vi "State_Machine.vi"(8 "error in (no error)":errorcluster caption="entrée d'erreur (pas d'erreur)", 11 "Get_Voltage en entrée":refnum<class "Nodon_Generate_SN.lvclass">) -> (0 "error out":errorcluster caption="sortie d'erreur", 2 "Json_String":string, 3 "Get_Voltage en sortie":refnum<class "Nodon_Generate_SN.lvclass">)   [LabVIEW 2020, in "Library Test.lvlib" / "Nodon_Generate_SN.lvclass"]
uses:
  Nodon_Generate_SN.lvclass
  E:/Dev/SVN TB45/TB45/Class/Test/Test (Default)/Test (Default).lvclass
  Database/Database Altyor/Database Altyor.lvclass
  E:/Dev/SVN TB45/TB45/Class/Database/Database drivers/Database Drivers.lvclass
  JSON API/JSON Value/Set from JSON string.vi
  Instrument/Instrument (Default)/Class Instrument (Default).lvclass
  JSON API/JSON Value/JSON Value.lvclass
  Nodon_Generate_SN.lvclass/Nodon_Generate_SN.ctl
  JSON API/Variant JSON/Variant JSON.lvlib
  JSON API/Get Polymorphic/JSON GetSet.lvlib
  Commun VI/Library Commun.lvlib
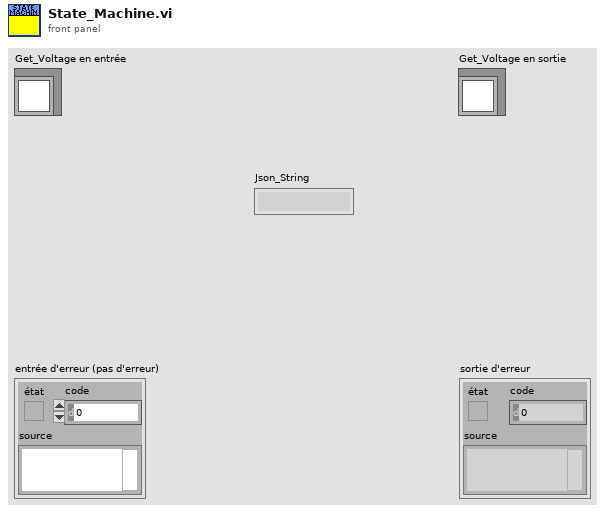
[diagram p1: front panel]
types:
  T1 = cluster{"Connection Name ODBC":string, "DatabaseName":string, "Condition":string, "Type Data ":enum16{"Data Product", "Data Test"}, "Database Altyor":refnum<class "Database Altyor.lvclass">}
  T2 = cluster{"idTest":u32, "CreationDate":string, "EndOfProduction":string, "OrderNumber":string, "Batch":string, "ProductName":string, "PartNumber":string, "SerialNumber":string, "Operator":string, "Result":string, "AdditionalInformation":string}[]
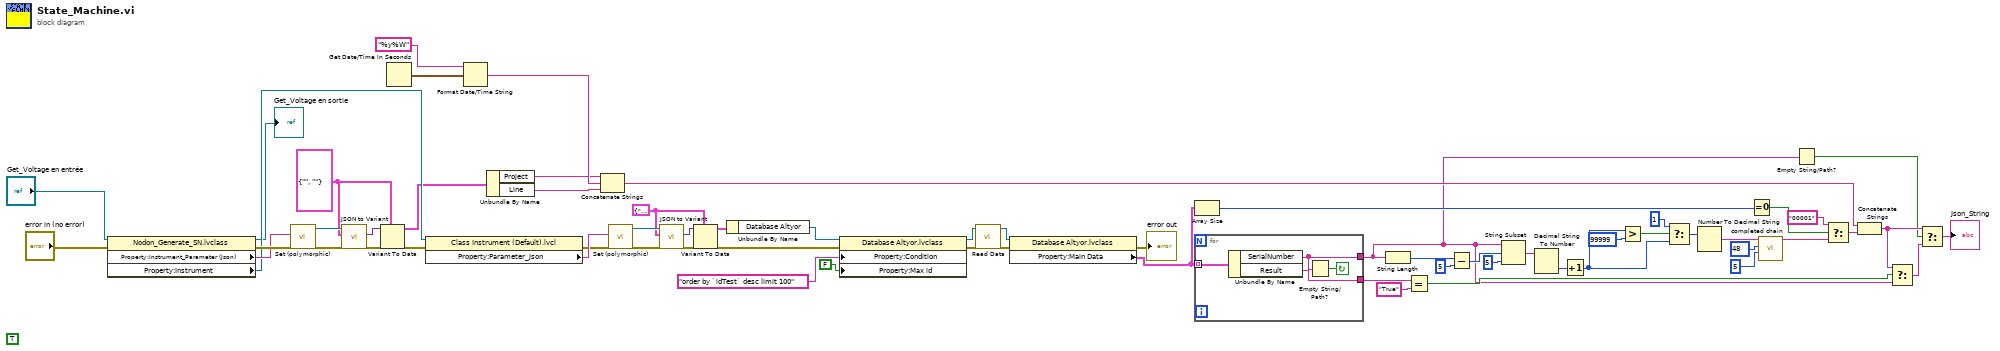
[diagram p0: block diagram]
diagram:
  (unwired) TRUE ("Max id")
  w48 = cluster{"Project":string, "Line":string} {"Project"="", "Line"=""}
  w60 = T1 {"Connection Name ODBC"="", "DatabaseName"="", "Condition"="", "Type Data "=enum."Data Product", "Database Altyor"=refnum} ("Parameter")
  n1 = property class="Nodon_Generate_SN.lvclass"(reference="Get_Voltage en entrée", error in="error in (no error)") -> (reference out=→"Get_Voltage en sortie":refnum<class "Nodon_Generate_SN.lvclass">, error out=w52:errorcluster, "Property:Instrument_Parameter (Json)"=w51:string, "Property:Instrument"=w47:refnum<class "Class Instrument (Default).lvclass">)
  n2 = call-poly "Set (polymorphic).vi"("error in (no error)"=w52, "JSON stream"=w51) -> ("error out"=w54:errorcluster, "JSON Value out"=w56:refnum<class "JSON Value.lvclass">)  [unwired: 7 in, 1 out]
  n3 = call "JSON to Variant.vi"("error in (no error)"=w54, "Variant (Data Type)"=w48, "JSON Value"=w56) -> ("error out"=w55:errorcluster, "Variant out"=w53:variant)  [unwired: 7 in]
  n4 = Variant To Data(error in=w55, type=w48, Variant=w53) -> (data=w42:cluster{"Project":string, "Line":string}, error out=w46:errorcluster)
  n5 = Get Date/Time In Seconds() -> (seconds since 1Jan1904=w45:timestamp)
  n6 = property class="Class Instrument (Default).lvcl"(reference=w47, error in=w46) -> (error out=w58:errorcluster, "Property:Parameter_Json"=w59:string)  [unwired: 1 out]
  n7 = Format Date/Time String(time format string (%c)="%y%W" ("chaîne de format de l'heure (%c)"), seconds (now)=w45) -> (date/time string=w43:string)  [unwired: 1 in]
  n8 = Unbundle By Name(w42) -> ("Project"=w41:string, "Line"=w40:string)
  n9 = Concatenate Strings(w41, w43, w40) -> (w18:string)
  n10 = call-poly "Set (polymorphic).vi"("error in (no error)"=w58, "JSON stream"=w59) -> ("error out"=w62:errorcluster, "JSON Value out"=w64:refnum<class "JSON Value.lvclass">)  [unwired: 7 in, 1 out]
  n11 = call "JSON to Variant.vi"("error in (no error)"=w62, "Variant (Data Type)"=w60, "JSON Value"=w64) -> ("error out"=w63:errorcluster, "Variant out"=w61:variant)  [unwired: 7 in]
  n12 = Variant To Data(error in=w63, type=w60, Variant=w61) -> (data=w57:T1, error out=w12:errorcluster)
  n13 = Unbundle By Name(w57) -> ("Database Altyor"=w11:refnum<class "Database Altyor.lvclass">)
  n14 = property class="Database Altyor.lvclass"(reference=w11, error in=w12, "Property:Condition"="order by `idTest` desc limit 100" ("chaîne"), "Property:Max id"=FALSE ("Max id")) -> (reference out=w23:refnum<class "Database Altyor.lvclass">, error out=w22:errorcluster)
  n15 = call-dynamic "Read Data.vi"("error in (no error)"=w22, "Database Altyor en entrée"=w23) -> ("error out"=w20:errorcluster, "Database Altyor en sortie"=w21:refnum<class "Database Altyor.lvclass">)  [unwired: 8 in]
  n16 = property class="Database Altyor.lvclass"(reference=w21, error in=w20) -> (error out=→"error out":errorcluster, "Property:Main Data"=w10:T2)  [unwired: 1 out]
  n17 = Array Size(array=w10) -> (size(s)=w9:i32)
  n18 = for {
    tunnel: w10 -> [w68] mode=indexing
    tunnel: [w67] -> w8
    tunnel: [w66] -> w2
    stop <- w65 continue-if-true
    n19 = Unbundle By Name(w68) -> ("SerialNumber"=w66:string, "Result"=w67:string)
    n20 = Empty String/Path?(string/path=w66) -> (empty?=w65:bool)
  }
  n21 = String Length(string=w2) -> (length=w38:i32)
  n22 = Equal?(x=w8, y="True") -> (x = y?=w15:bool)
  n23 = Subtract(x=w38, y=5 ("x")) -> (x-y=w37:i32)
  n24 = String Subset(string=w2, offset (0)=w37, length (rest)=5 ("longueur (reste)")) -> (substring=w31:string)
  n25 = Decimal String To Number(string=w31) -> (number=w30:i32)  [unwired: 2 in, 1 out]
  n26 = Increment(x=w30) -> (x+1=w26:i32)
  n27 = Greater?(x=w26, y=99999) -> (0:w28:bool)
  n28 = Select(t=1 ("y"), s=w28, f=w26) -> (s? t:f=w25:i32)
  n29 = Number To Decimal String(number=w25) -> (decimal integer string=w34:string)  [unwired: 1 in]
  n30 = Equal To 0?(x=w9) -> (x = 0?=w6:bool)
  n31 = call "completed chain.vi"("longueur"=5, "Combler par"=u8 48, "Chaine"=w34) -> ("chaîne"=w16:string)  [unwired: 8 in]
  n32 = Empty String/Path?(string/path=w2) -> (empty?=w1:bool)
  n33 = Select(t="00001" ("cas vrai"), s=w6, f=w16) -> (s? t:f=w24:string)
  n34 = Concatenate Strings(w18, w24) -> (w5:string)
  n35 = Select(t=w5, s=w15, f=w2) -> (s? t:f=w4:string)
  n36 = Select(t=w5, s=w1, f=w4) -> (s? t:f=→"Json_String":string)
